vi "SubVI_CinematicaInversa.vi"(0 "Posição desejada (x,y,z)":dbl[](array[numeric]), 1 "Posição desejada (roll, pitch, yaw)":dbl[](array[numeric]), 2 "Posição atual (juntas)":dbl[](array[numeric])) -> (7 "Posição desejada (juntas)":dbl[](array[numeric]), 10 "error out":errorcluster)   [LabVIEW 2017]
uses:
  <vilib>/Analysis/coordinate.llb/Angle Units.ctl
  <vilib>/Analysis/coordinate.llb/Angle Range (Degree).ctl
  <vilib>/Analysis/coordinate.llb/Wrap Angle (array).vi
  <vilib>/Analysis/coordinate.llb/Wrap Angle (scalar).vi
  <vilib>/robotics/Kinematics/RotateX.vi
  <vilib>/robotics/Kinematics/RotateY.vi
  <vilib>/robotics/Kinematics/RotateZ.vi
  <vilib>/Analysis/baseanly.llb/A x B.vi
  <vilib>/Analysis/baseanly.llb/Real A x B.vi
  <vilib>/robotics/Kinematics/Robot/Inverse Kinematics (Point).vi
  <vilib>/picture/3D Picture Control/Object/Add Object (reference).vi
  <vilib>/imath/engines/lvmath2/RunTimeEngine/Managers/WorkSpace/UID Generator.vi
  <vilib>/imath/engines/lvmath2/RunTimeEngine/BuiltInFunctions/asin/NIMS_asin(C).vi
  <instcachedir>/0/NIMS_asin(C)_AC3BFCB47B1546A49EF59786BF54013C.lvgen/NIMS_asin(C)_AC3BFCB47B1546A49EF59786BF54013C_001.vi
  <vilib>/imath/engines/lvmath2/RunTimeEngine/ArithmeticOperatorToken/NIMS_ArithmeticOperator_power(S).vi
  <instcachedir>/0/NIMS_ArithmeticOperator_power(S)_86B1D76B77564424912EAFCCCC7488ED.lvgen/NIMS_ArithmeticOperator_power(S)_86B1D76B77564424912EAFCCCC7488ED_010.vi
  <vilib>/imath/engines/lvmath2/RunTimeEngine/BuiltInFunctions/acos/NIMS_acos(C).vi
  <instcachedir>/0/NIMS_acos(C)_09AB0EA1D77D44F8AD620F57E6E2841E.lvgen/NIMS_acos(C)_09AB0EA1D77D44F8AD620F57E6E2841E_001.vi
  <vilib>/imathl/engines/lvmath/Functions/Error Handling/Create Error.vi
  <vilib>/imath/engines/lvmath2/RunTimeEngine/BuiltInFunctions/sin/NIMS_sin(C).vi
  <instcachedir>/0/NIMS_sin(C)_3AEF00A0D47841AA8A3F5FC7392BEEFD.lvgen/NIMS_sin(C)_3AEF00A0D47841AA8A3F5FC7392BEEFD_001.vi
  <vilib>/imath/engines/lvmath2/RunTimeEngine/RunTimeType/NIMS_RunTimeType_From StrictType (excl LVString).vi
  <instcachedir>/0/NIMS_RunTimeType_From StrictType (excl LVString)_1019F277F0A747EDBCA0F6C52CA54500.lvgen/NIMS_RunTimeType_From StrictType (excl LVString)_1019F277F0A747EDBCA0F6C52CA54500_000.vi
  <vilib>/imath/engines/lvmath2/RunTimeEngine/LocalVariableDefStatement/MC_LocalVariableDefStatement_Display.vi
  <vilib>/imath/engines/lvmath2/RunTimeEngine/IndexReplace/NIMS V(S)=S.vi
  <instcachedir>/0/NIMS V(S)=S_3F4D177D41884A9C969E5FA0B22E4B28.lvgen/NIMS V(S)=S_3F4D177D41884A9C969E5FA0B22E4B28_003.vi
  <vilib>/imath/engines/lvmath2/RunTimeEngine/IndexRead/NIMS V(S).vi
  <instcachedir>/0/NIMS V(S)_0488751826AF41519A22953C041130DC.lvgen/NIMS V(S)_0488751826AF41519A22953C041130DC_002.vi
  <instcachedir>/0/NIMS V(S)=S_3F4D177D41884A9C969E5FA0B22E4B28.lvgen/NIMS V(S)=S_3F4D177D41884A9C969E5FA0B22E4B28_000.vi
  <vilib>/imath/engines/lvmath2/RunTimeEngine/ErrorHandling/NIMS_Create Error From Enums.vi
  <instcachedir>/0/NIMS V(S)_0488751826AF41519A22953C041130DC.lvgen/NIMS V(S)_0488751826AF41519A22953C041130DC_000.vi
  <vilib>/imath/engines/lvmath2/RunTimeEngine/BuiltInFunctions/cos/NIMS_cos(C).vi
  <instcachedir>/0/NIMS_cos(C)_D76AB42705D04DD7AB90183D51B32C21.lvgen/NIMS_cos(C)_D76AB42705D04DD7AB90183D51B32C21_001.vi
  <instcachedir>/0/NIMS V(S)=S_3F4D177D41884A9C969E5FA0B22E4B28.lvgen/NIMS V(S)=S_3F4D177D41884A9C969E5FA0B22E4B28_001.vi
  <instcachedir>/0/NIMS V(S)_0488751826AF41519A22953C041130DC.lvgen/NIMS V(S)_0488751826AF41519A22953C041130DC_003.vi
  <vilib>/imath/engines/lvmath2/RunTimeEngine/Managers/SymbolTable/Clear UID.vi
  <vilib>/imath/engines/lvmath2/RunTimeEngine/NodeEndStatement/NIMS_NodeEndStatement_Output.vi
  <instcachedir>/0/NIMS_NodeEndStatement_Output_53EC0D466D134D7ABD903AC30B43404B.lvgen/NIMS_NodeEndStatement_Output_53EC0D466D134D7ABD903AC30B43404B_000.vi
  <instcachedir>/0/NIMS_NodeEndStatement_Output_53EC0D466D134D7ABD903AC30B43404B.lvgen/NIMS_NodeEndStatement_Output_53EC0D466D134D7ABD903AC30B43404B_009.vi
  <vilib>/imath/engines/lvmath2/RunTimeEngine/ErrorHandling/NIMS_Finalize Error.vi
  <vilib>/robotics/Kinematics/Plotting/NI_Robotics_3DKinematics.lvlib
  <vilib>/picture/3D Picture Control/NI_3D Picture Control.lvlib
  <vilib>/robotics/Kinematics/NI_Kinematics.lvlib
  <vilib>/Analysis/NI_AAL_Angle.lvlib
  <vilib>/imath/engines/lvmath2/RunTimeEngine/Managers/SymbolTable/NIMS_WorkSpace.lvlib
panel:
  out "angle out":dbl
  out "Posição":cluster{"X":dbl[], "Y":dbl[]}(graph)
  out "3D Picture Control":refnum<vi>(3d-picture)
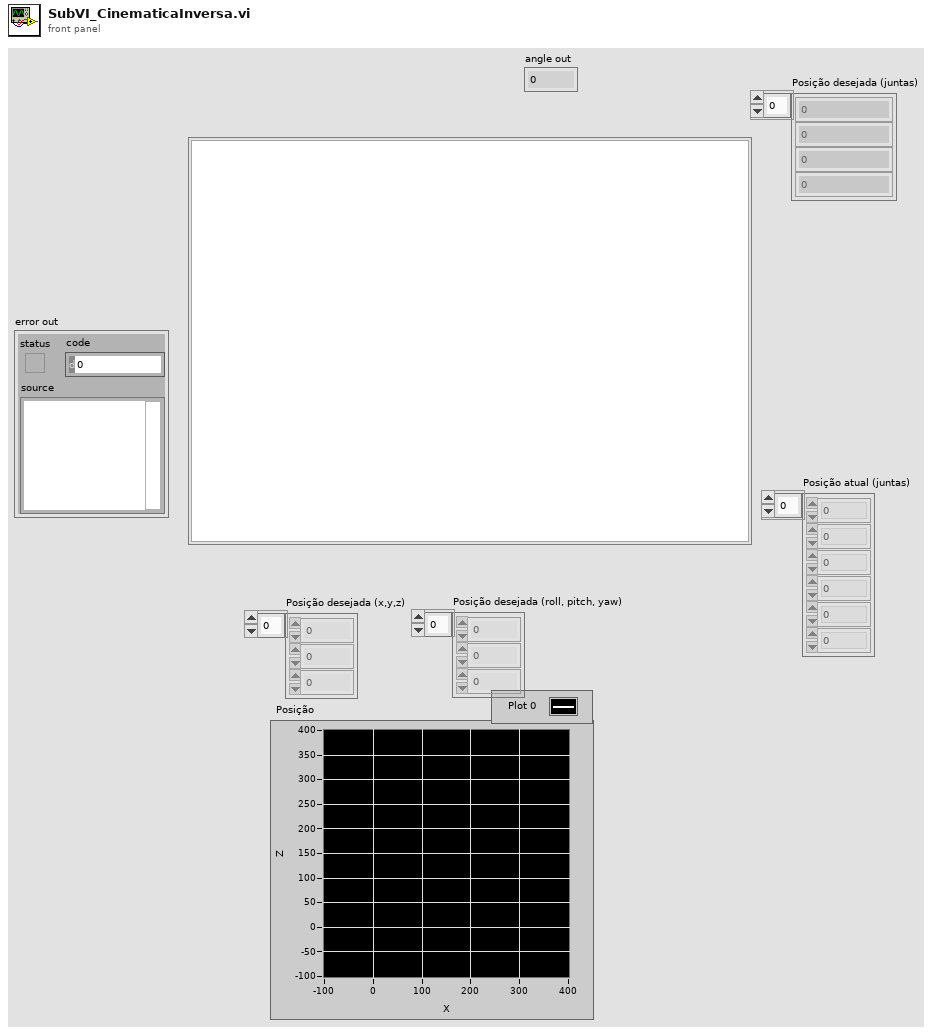
[diagram p1: front panel]
types:
  T1 = typedef "NI_AAL_Angle.lvlib/Angle Range (Degree).ctl" = u16
  T2 = typedef "NI_AAL_Angle.lvlib/Angle Units.ctl" = i32
  T3 = cluster{"Numeric":dbl, "Numeric":dbl, "Numeric":dbl}
  T4 = typedef "NI_Matrix.lvlib/RealMatrix.ctl" = dbl[][]
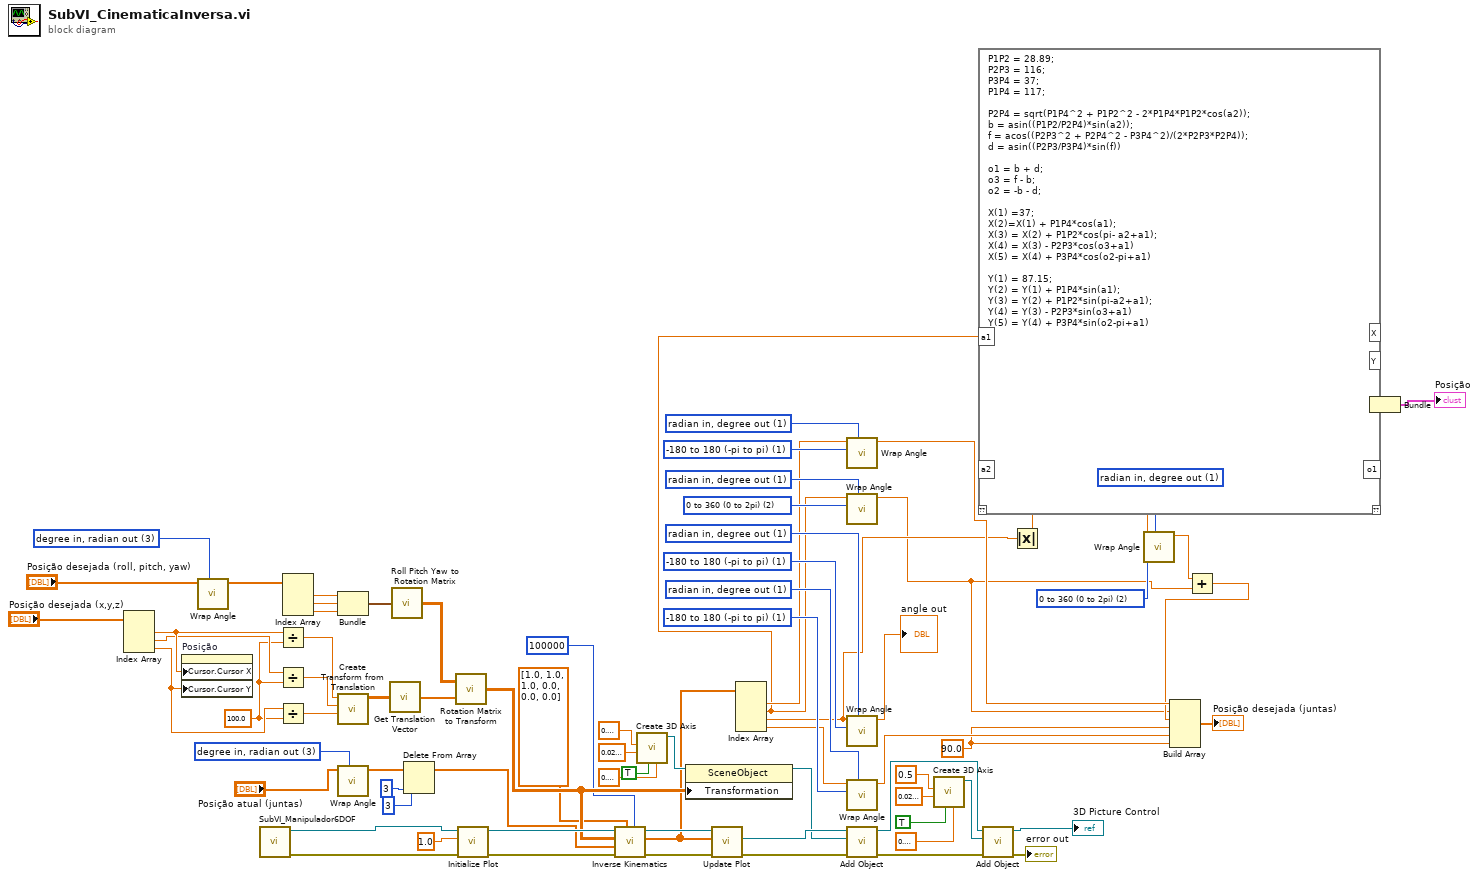
[diagram p0: block diagram]
diagram:
  w13 = T1 2 items=["none", "-180 to 180 (-pi to pi)", "0 to 360 (0 to 2pi)"] ("angle range")
  w14 = T2 1 items=["radian in, radian out", "radian in, degree out", "degree in, degree out", "degree in, radian out"] ("angle units")
  w18 = 90.0 ("element")
  w24 = T2 1 items=["radian in, radian out", "radian in, degree out", "degree in, degree out", "degree in, radian out"] ("angle units")
  w23 = T1 1 items=["none", "-180 to 180 (-pi to pi)", "0 to 360 (0 to 2pi)"] ("angle range")
  w25 = T2 1 items=["radian in, radian out", "radian in, degree out", "degree in, degree out", "degree in, radian out"] ("angle units")
  w26 = T1 1 items=["none", "-180 to 180 (-pi to pi)", "0 to 360 (0 to 2pi)"] ("angle range")
  w28 = T2 1 items=["radian in, radian out", "radian in, degree out", "degree in, degree out", "degree in, radian out"] ("angle units")
  w27 = T1 2 items=["none", "-180 to 180 (-pi to pi)", "0 to 360 (0 to 2pi)"] ("angle range")
  w32 = T2 3 items=["radian in, radian out", "radian in, degree out", "degree in, degree out", "degree in, radian out"] ("angle units")
  w34 = T2 3 items=["radian in, radian out", "radian in, degree out", "degree in, degree out", "degree in, radian out"] ("angle units")
  w38 = T2 1 items=["radian in, radian out", "radian in, degree out", "degree in, degree out", "degree in, radian out"] ("angle units")
  w39 = T1 1 items=["none", "-180 to 180 (-pi to pi)", "0 to 360 (0 to 2pi)"] ("angle range")
  w41 = 100.0 ("y")
  n1 = Index Array(array="Posição desejada (x,y,z)") -> (element #1=w47:dbl, element #2=w42:dbl, element #3=w46:dbl)  [unwired: 3 in]
  n2 = property on="Posição" class="XYGraph (strict)"("Cursor.Cursor X"=w47, "Cursor.Cursor Y"=w46) -> ()  [unwired: 2 in, 2 out]
  n3 = call-poly <vilib>:"Wrap Angle.vi"("angle units"=w34, "Angle In"="Posição desejada (roll, pitch, yaw)") -> ("Angle Out"=w35:dbl[])  [unwired: 8 in, 1 out]
  n4 = call "SubVI_Manipulador6DOF.vi"() -> ("error out"=w78:errorcluster, "NI_Robotics_Serial Robot Arm out"=w79:refnum<class "NI_Robotics_Serial Robot Arm.lvclass">)  [unwired: 10 in]
  n5 = Divide(x=w47, y=w41) -> (x/y=w50:dbl)
  n6 = Divide(x=w42, y=w41) -> (x/y=w40:dbl)
  n7 = Divide(x=w46, y=w41) -> (x/y=w49:dbl)
  n8 = Index Array(array=w35) -> (element #1=w45:dbl, element #2=w44:dbl, element #3=w43:dbl)  [unwired: 3 in]
  n9 = Bundle("Numeric"=w45, "Numeric"=w44, "Numeric"=w43) -> (w37:T3)  [unwired: 1 in]
  n10 = call <vilib>:"Create Transform from Translation.vi"("z"=w49, "y"=w40, "x"=w50) -> ("transform"=w58:T4)  [unwired: 8 in]
  n11 = call-poly <vilib>:"Wrap Angle.vi"("angle units"=w32, "Angle In"="Posição atual (juntas)") -> ("Angle Out"=w31:dbl[])  [unwired: 8 in, 1 out]
  n12 = call <vilib>:"Get Translation Vector.vi"("transform"=w58) -> ("translation vector"=w57:dbl[])
  n13 = call <vilib>:"Roll Pitch Yaw to Rotation Matrix.vi"("angles"=w37) -> ("rotation matrix"=w59:T4)
  n14 = Delete From Array(array=w31, length=3, index=3) -> (array with subset deleted=w10:dbl[])  [unwired: 1 out]
  n15 = call <vilib>:"Rotation Matrix to Transform.vi"("translation vector"=w57, "rotation matrix"=w59) -> ("transform"=w56:T4)
  n16 = call <vilib>:"Initialize Plot.vi"("error in (no error)"=w78, "scale (1)"=1.0, "serial arm in"=w79) -> ("error out"=w73:errorcluster, "serial arm out"=w71:refnum<class "NI_Robotics_Serial Robot Arm.lvclass">)  [unwired: 7 in]
  n17 = call-poly <vilib>:"Inverse Kinematics.vi"("max steps"=100000, "mask"=dbl[] [1.0, 1.0, 1.0, 0.0, 0.0, 0.0], "error in (no error)"=w73, "current joint positions"=w10, "end effector transform"=w56, "serial arm in"=w71) -> ("error out"=w61:errorcluster, "joint positions"=w29:dbl[], "serial arm out"=w60:refnum<class "NI_Robotics_Serial Robot Arm.lvclass">)  [unwired: 2 in, 1 out]
  n18 = call <vilib>:"Create 3D Axis.vi"("Character Size"=sgl 0.2, "Axis label?"=TRUE, "Radius"=sgl 0.03, "Length"=sgl 0.2) -> ("New Object Refnum"=w70:refnum<vi>)  [unwired: 6 in, 1 out]
  n19 = property class="SceneObject"(reference=w70, "Transformation"=w56) -> (reference out=w62:refnum<vi>)  [unwired: 1 in, 1 out]
  n20 = call <vilib>:"Update Plot.vi"("error in (no error)"=w61, "joint positions"=w29, "serial arm in"=w60) -> ("error out"=w64:errorcluster, "serial arm scene"=w63:refnum<vi>)  [unwired: 6 in, 1 out]
  n21 = Index Array(array=w29) -> (element #1=w22:dbl, element #2=w2:dbl, element #3=w4:dbl, element #4=w20:dbl)  [unwired: 4 in]
  n22 = call-poly <vilib>:"Wrap Angle.vi"("angle units"=w38, "angle range"=w39, "angle in"=w22) -> ("angle out"=w21:dbl)  [unwired: 7 in, 1 out]
  n23 = call-poly <vilib>:"Wrap Angle.vi"("angle units"=w28, "angle range"=w27, "angle in"=w2) -> ("angle out"=w1:dbl)  [unwired: 7 in, 1 out]
  n24 = call-poly <vilib>:"Wrap Angle.vi"("angle units"=w25, "angle range"=w26, "angle in"=w4) -> ("angle out"=→"angle out":dbl)  [unwired: 7 in, 1 out]
  n25 = call-poly <vilib>:"Wrap Angle.vi"("angle units"=w24, "angle range"=w23, "angle in"=w20) -> ("angle out"=w19:dbl)  [unwired: 7 in, 1 out]
  n26 = call-poly <vilib>:"Add Object.vi"("error in (no error)"=w64, "New Object In"=w62, "Scene Object In"=w63) -> ("error out"=w54:errorcluster, "Scene Object Out"=w53:refnum<vi>)  [unwired: 6 in, 1 out]
  n27 = call <vilib>:"Create 3D Axis.vi"("Character Size"=sgl 0.2, "Axis label?"=TRUE, "Radius"=sgl 0.03, "Length"=sgl 0.5) -> ("New Object Refnum"=w65:refnum<vi>)  [unwired: 6 in, 1 out]
  n28 = call-poly <vilib>:"Add Object.vi"("error in (no error)"=w54, "New Object In"=w65, "Scene Object In"=w53) -> ("error out"=→"error out":errorcluster, "Scene Object Out"=→"3D Picture Control":refnum<vi>)  [unwired: 6 in, 1 out]
  n29 = Absolute Value(x=w4) -> (abs(x)=w16:dbl)
  n30 = mathscript code="P1P2 = 28.89;\nP2P3 = 116;\nP3P4 = 37;\nP1P4 = 117;\n\nP2P4 = sqrt(P1P4^2 + P1P2^2 - 2*P1P4*P1P2*cos(a2));\nb = asin((P1P2/P2P4)*sin(a2));\nf = acos((P2P3^2 + P2P4^2 - P3P4^2)/(2*P2P3*P2P4));\nd = asin((P2P3/P3P4)*sin(f))\n\no1 = b + d;\no3 = f - b;\no2 = -b - d;\n\nX(1) =37;\nX(2)=X(1) + P1P4*cos(a1);\nX(3) = X(2) + P1P2*cos(pi- a2+a1);\nX(4) = X(3) - P2P3*cos(o3+a1)\nX(5) = X(4) + P3P4*cos(o2-pi+a1)\n\nY(1) = 87.15;\nY(2) = Y(1) + P1P4*sin(a1);\nY(3) = Y(2) + P1P2*sin(pi-a2+a1);\nY(4) = Y(3) - P2P3*sin(o3+a1)\nY(5) = Y(4) + P3P4*sin(o2-pi+a1)"("a2"=w16, "a1"=w2) -> ("o1"=w15:cdb, "X"=w6:cdb[], "Y"=w5:cdb[])  [unwired: 1 in, 1 out]
  n31 = call-poly <vilib>:"Wrap Angle.vi"("angle units"=w14, "angle range"=w13, "angle in"=w15) -> ("angle out"=w12:dbl)  [unwired: 7 in, 1 out]
  n32 = Add(x=w12, y=w1) -> (x+y=w11:dbl)
  n33 = Build Array(w21, w1, w11, w18, w19, w18) -> (→"Posição desejada (juntas)":dbl[])
  n34 = Bundle("X"=w6, "Y"=w5) -> (→"Posição":cluster{"X":cdb[], "Y":cdb[]})  [unwired: 1 in]
